vi "2015Swerve_SteeringAdjustment.vi"(9 "Wheel Power":dbl, 10 "Encoder Setpoint":dbl, 11 "Encoder Position":dbl) -> (1 "Wheel Power Out":dbl, 2 "Encoder Setpoint Out":dbl)   [LabVIEW 2014]
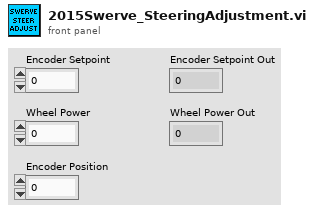
[diagram p1: front panel]
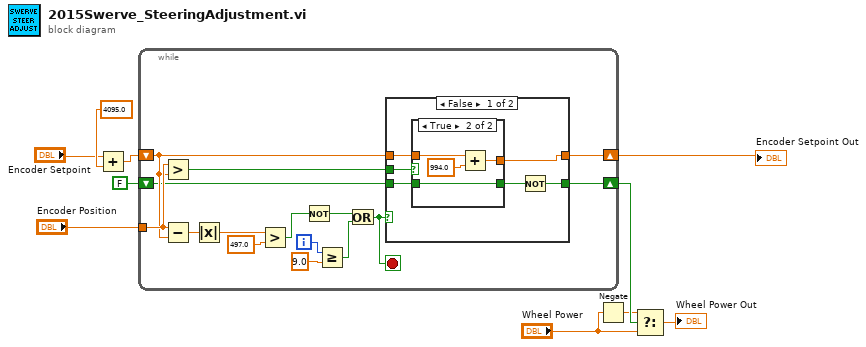
[diagram p0: block diagram]
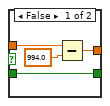
[diagram p2: hidden frame]
diagram:
  n1 = Add(x="Encoder Setpoint", y=4095.0) -> (x+y=w2:dbl)
  n2 = while {
    tunnel: "Encoder Position" -> [w15]
    shift-right: [w22] -> w1
    shift-left: w2 -> [w14]
    shift-right: [w12] -> w8
    shift-left: FALSE -> [w11]
    i -> [w23]
    stop <- w13 stop-if-true
    n3 = Greater?(x=w15, y=w14) -> (0:w16:bool)
    n4 = Subtract(x=w15, y=w14) -> (x-y=w20:dbl)
    n5 = Absolute Value(x=w20) -> (abs(x)=w19:dbl)
    n6 = Greater?(x=w19, y=497.0) -> (0:w18:bool)
    n7 = Not(x=w18) -> (.not. x?=w17:bool)
    n8 = Greater Or Equal?(x=w23, y=9.0) -> (x >= y?=w25:bool)
    n9 = Or(x=w17, y=w25) -> (x .or. y?=w13:bool)
    n10 = case shown="False" w13 {
      tunnel: [w31 w41] -> w22
      tunnel: w16 -> [w30 _]
      tunnel: w14 -> [w29 w41]
      tunnel: [w26 w40] -> w12
      tunnel: w11 -> [w27 w40]
      frame False {
        n11 = case shown="True" w30 {
          tunnel: w29 -> [w35 w39]
          tunnel: [w33 w37] -> w31
          tunnel: [w32 w36] -> w28
          tunnel: w27 -> [w32 w36]
          frame False {
            n12 = Subtract(x=w35, y=994.0) -> (x-y=w33:dbl)
          }
          frame True {
            n13 = Add(x=w39, y=994.0) -> (x+y=w37:dbl)
          }
        }
        n14 = Not(x=w28) -> (.not. x?=w26:bool)
      }
      frame True {
      }
    }
  }
  "Encoder Setpoint Out" <- w1
  n15 = Negate(x="Wheel Power") -> (-x=w7:dbl)
  n16 = Select(t=w7, s=w8, f="Wheel Power") -> (s? t:f=→"Wheel Power Out":dbl)
